vi "Robot Global Data.vi"() -> ()   [LabVIEW 2020]
doc: "This global VI can contain as many global variables as you need. Place a control on the panel, give it a good name. To read or write to it from a VI, drag the icon to the diagram of that VI. You can also drag from the project. Click on the node to change which global you access. You shouldn't have multiple locations writing to a global or it will cause a race-condition."
uses:
  <vilib>/Rock Robotics/WPI/Camera/WPI_CameraImageSize.ctl
  <vilib>/Rock Robotics/WPI/DriverStation/WPI_DriverStationRobotMode2.ctl
  <vilib>/Rock Robotics/WPI/ThirdParty/JAS_Junk/TrajLib/TypeDef/POSE2D.ctl
  <vilib>/Rock Robotics/WPI/ThirdParty/JAS_Junk/TrajLib/TypeDef/TRANSLATION2D.ctl
  <vilib>/Rock Robotics/WPI/ThirdParty/JAS_Junk/TrajLib/TypeDef/ROTATION2D.ctl
  <vilib>/Rock Robotics/WPI/ThirdParty/JAS_Junk/TrajLib/TypeDef/SWERVE_DRIVE_ODOMETRY.ctl
  <vilib>/Rock Robotics/WPI/ThirdParty/JAS_Junk/TrajLib/TypeDef/SWERVE_DRIVE_MODULE_POSITION.ctl
  <vilib>/Rock Robotics/WPI/ThirdParty/JAS_Junk/TrajLib/Trajectory_Library.lvlib
panel:
  in  "AutoState":string
  out "Home2":bool
  in  "Escalator Pid":bool
  out "Escalator Set":dbl
  out "Escalator Enc":dbl
  out "Elevator Off Set":dbl
  out "POV2":i16=-1
  out "RStick2":bool
  out "LStick2":bool
  out "Option2":bool
  out "Share2":bool
  out "RightBumper2":bool
  out "LeftBumper2":bool
  out "X2":bool
  out "Circle2":bool
  out "Triangle2":bool
  out "Square2":bool
  out "RightTrigger2":dbl
  out "LeftTrigger2":dbl
  out "RightY2":dbl
  out "RightX2":dbl
  out "LeftY2":dbl
  out "LeftX2":dbl
  out "Tz":dbl
  out "Tx":dbl
  out "YawReset":bool
  out "ENCreset":bool
  out "OdometerReset":bool
  out "SWERVE_DRIVE_ODOMETRY":T1={"POSE"={"TRANSLATION"={"X"=0.0, "Y"=0.0}, "ROTATION"={"VALUE"=0.0, "COS"=1.0, "SIN"=0.0}}, "GyroOffset"={"VALUE"=0.0, "COS"=1.0, "SIN"=0.0}, "PreviousAngle"={"VALUE"=0.0, "COS"=1.0, "SIN"=0.0}, "PrevModulePositions"=[], "NumModules"=0} {"PrevModulePositions"."Angle"."SIN" format="%13.4f"; "PrevModulePositions"."Angle"."COS" format="%13.4f"; "PrevModulePositions"."Angle"."VALUE" format="%13.4f"; "PreviousAngle"."SIN" format="%13.4f"; "PreviousAngle"."COS" format="%13.4f"; "PreviousAngle"."VALUE" format="%13.4f"; "GyroOffset"."SIN" format="%13.4f"; "GyroOffset"."COS" format="%13.4f"; "GyroOffset"."VALUE" format="%13.4f"; "POSE"."ROTATION"."SIN" format="%13.4f"; "POSE"."ROTATION"."COS" format="%13.4f"; "POSE"."ROTATION"."VALUE" format="%13.4f"; "POSE"."TRANSLATION"."Y" format="%14.3f"; "POSE"."TRANSLATION"."X" format="%14.3f"}
  out "Gravity Vector":cluster{"X":dbl, "Y":dbl, "Z":dbl}
  out "Enc3v":dbl
  out "Enc2v":dbl
  out "Enc1v":dbl
  out "Enc0v":dbl
  out "CSVerrr":bool
  out "robot POSE":T2={"TRANSLATION"={"X"=0.0, "Y"=0.0}, "ROTATION"={"VALUE"=0.0, "COS"=1.0, "SIN"=0.0}} {"ROTATION"."SIN" format="%13.4f"; "ROTATION"."COS" format="%13.4f"; "ROTATION"."VALUE" format="%13.4f"; "TRANSLATION"."Y" format="%14.3f"; "TRANSLATION"."X" format="%14.3f"}
  out "Az3":dbl
  out "Az2":dbl
  out "Az1":dbl
  out "Az0":dbl
  out "Roll":dbl
  out "Pitch":dbl
  out "Yaw":dbl
  out "Enc3d":dbl
  out "Enc2d":dbl
  out "Enc1d":dbl
  out "Enc0d":dbl
  out "Rumble":sgl
  out "POV1":i16=-1
  out "RStick1":bool
  out "LStick1":bool
  out "Option1":bool
  out "Share1":bool
  out "RightBumper1":bool
  out "LeftBumper1":bool
  out "X1":bool
  out "Circle1":bool
  out "Triangle1":bool
  out "Square1":bool
  out "RightTrigger1":dbl
  out "LeftTrigger1":dbl
  out "RightY1":dbl
  out "RightX1":dbl
  out "LeftY1":dbl
  out "LeftX1":dbl
  in  "Robot Mode":T6
  in  "image size":T7=enum."320x240"
  in  "Enable Vision":bool
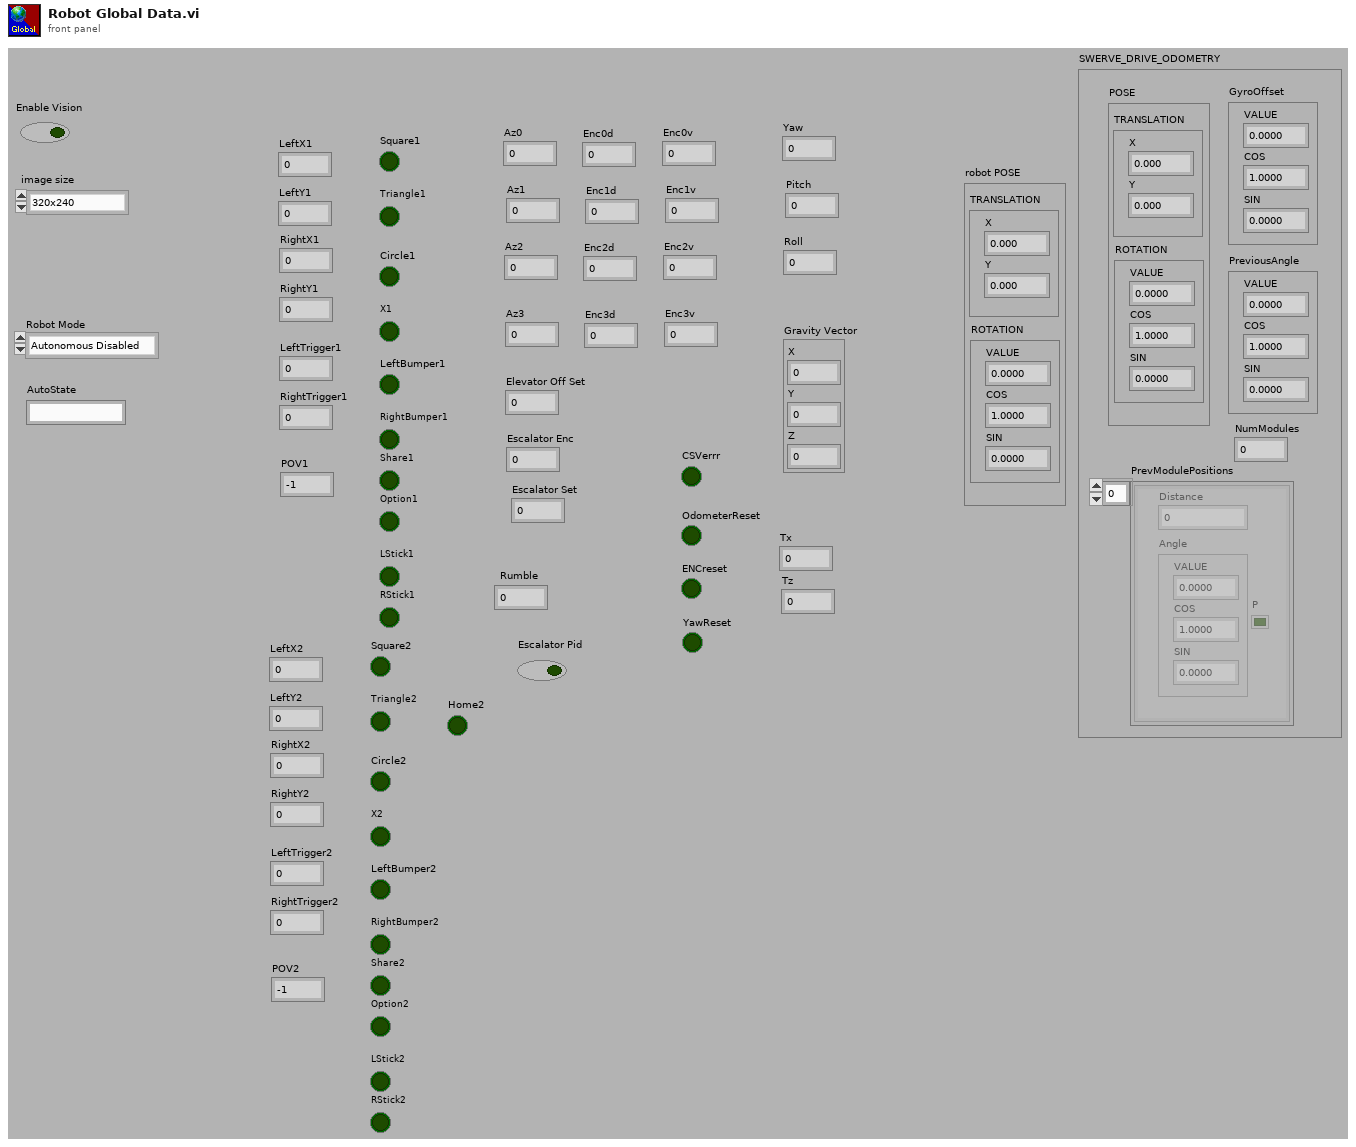
[diagram p1: front panel]
types:
  T1 = typedef "Trajectory_Library.lvlib/SWERVE_DRIVE_ODOMETRY.ctl" = cluster{"POSE":T2, "GyroOffset":T4, "PreviousAngle":T4, "PrevModulePositions":T5[], "NumModules":i32}
  T2 = typedef "Trajectory_Library.lvlib/POSE2D.ctl" = cluster{"TRANSLATION":T3, "ROTATION":T4}
  T3 = typedef "Trajectory_Library.lvlib/TRANSLATION2D.ctl" = cluster{"X":dbl, "Y":dbl}
  T4 = typedef "Trajectory_Library.lvlib/ROTATION2D.ctl" = cluster{"VALUE":dbl, "COS":dbl, "SIN":dbl}
  T5 = typedef "Trajectory_Library.lvlib/SWERVE_DRIVE_MODULE_POSITION.ctl" = cluster{"Distance":dbl, "Angle":T4, "P":bool}
  T6 = typedef "WPI_DriverStationRobotMode2.ctl" = enum16{"Autonomous Disabled", "Autonomous Enabled", "Teleop Disabled", "Teleop Enabled", "Disconnected", "Finish", "Test Disabled", "Test Enabled", "Emergency Stopped"}
  T7 = typedef "WPI_CameraImageSize.ctl" = enum16{"640x480", "320x240", "160x120", "Custom"}
diagram:
